vi "ConstellationRead.vi"(8 "error in":errorcluster, 9 "Active Boards":cluster{"Status":bool, "Board":string}[][](array[cluster]), 10 "Active Controllers":cluster{"Status":bool, "Number":dbl}[](array[cluster])=[{"Status"=TRUE, "Number"=0.0}, {"Status"=FALSE, "Number"=1.0}], 11 "Task in":refnum<visa-resource-name>[](array[refnum])) -> (0 "error out":errorcluster={"status"=FALSE, "code"=1073676294, "source"="VISA Read in ConstellationRead.vi->ConstellationTest.vi"}, 2 "Measurements":T1(array[cluster]), 3 "Task out":refnum<visa-resource-name>[](array[refnum]))   [LabVIEW 2012]
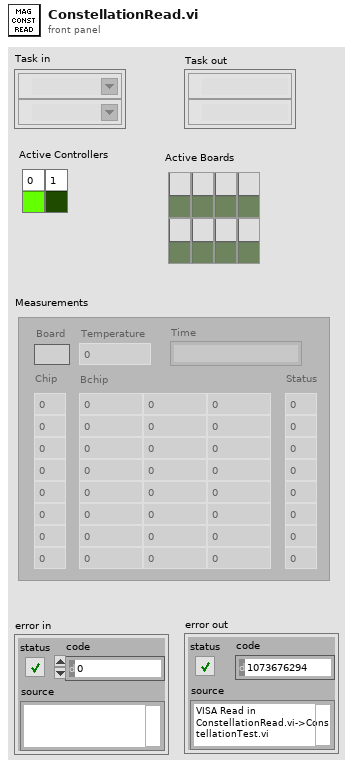
[diagram p1: front panel]
types:
  T1 = cluster{"Bchip":dbl[][], "Status":dbl[], "Temperature":dbl, "Chip":dbl[], "Board":string, "Time":string}[]
  T2 = cluster{"Bchip":dbl[][], "Status":dbl[], "Temperature":dbl, "Chip":dbl[], "Board":string, "Time Stamp":string}[]
  T3 = cluster{"Bchip":dbl[][], "Status":dbl[], "Temperature":dbl, "Chip":dbl[], "Board":string, "Time":string}
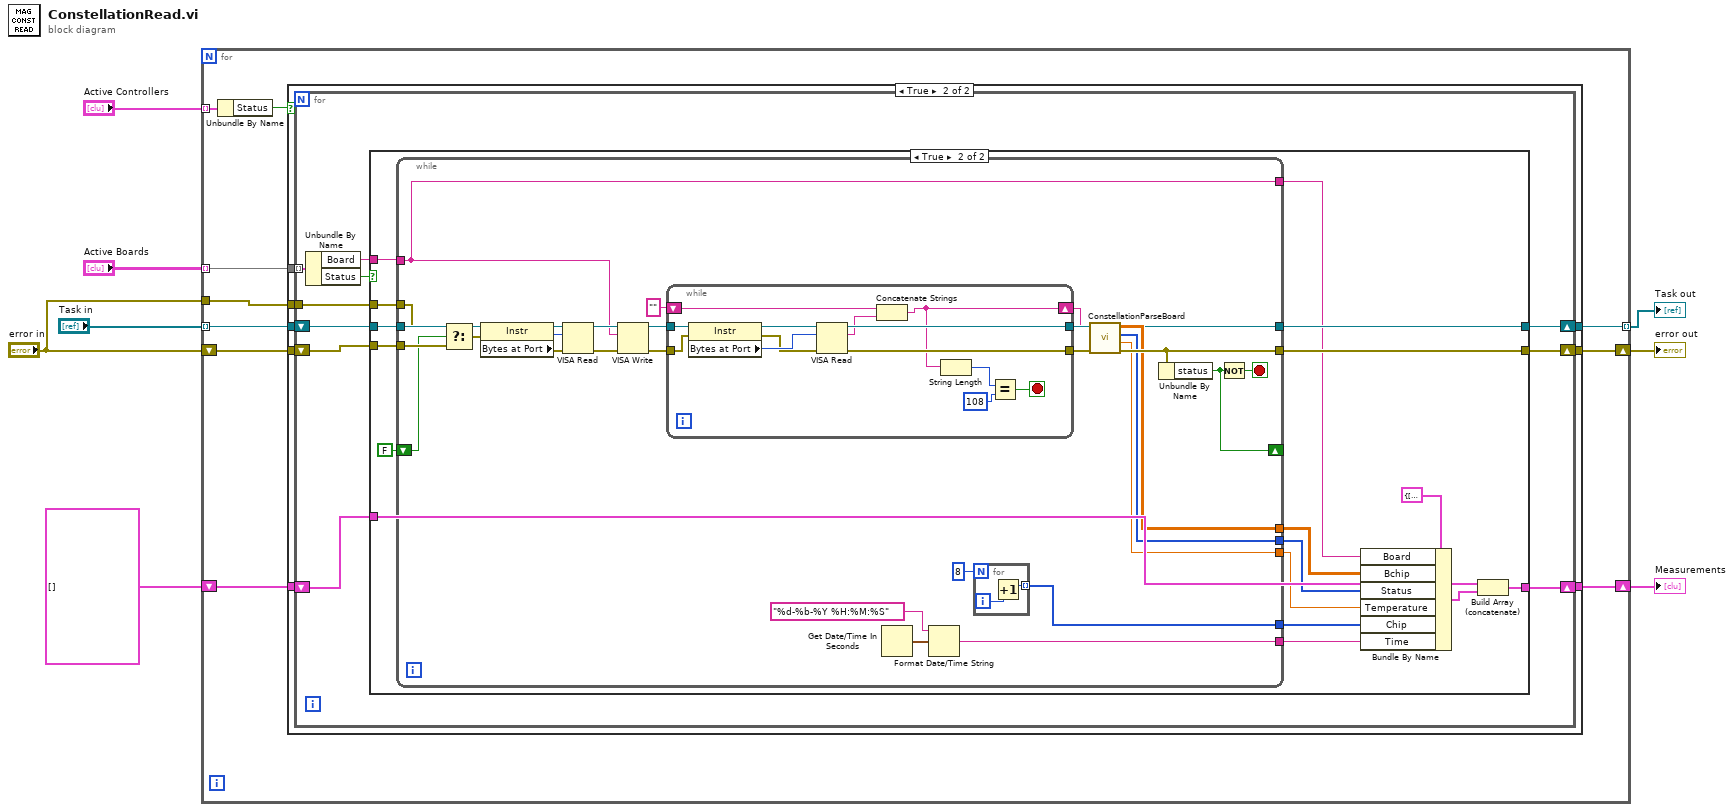
[diagram p0: block diagram]
diagram:
  n1 = for {
    tunnel: "Task in" -> [w16] mode=indexing
    tunnel: [w18] -> w6 mode=indexing
    shift-right: [w17] -> w7
    shift-left: "error in" -> [w15]
    tunnel: "error in" -> [w14]
    tunnel: "Active Controllers" -> [w13] mode=indexing
    shift-right: [w11] -> w3
    shift-left: T2 [] ("Measurements 2") -> [w10]
    tunnel: "Active Boards" -> [w9] mode=indexing
    n2 = Unbundle By Name(w13) -> ("Status"=w12:bool)
    n3 = case shown="True" w12 {
      tunnel: [w21 w29] -> w18
      tunnel: [w20 w28] -> w17
      tunnel: w16 -> [w21 w27]
      tunnel: w15 -> [w20 w26]
      tunnel: w14 -> [_ w25]
      tunnel: [w19 w24] -> w11
      tunnel: w10 -> [w19 w23]
      tunnel: w9 -> [_ w22]
      frame False {
      }
      frame True {
        n4 = for {
          shift-right: [w33] -> w29
          shift-left: w27 -> [w39]
          shift-right: [w34] -> w28
          shift-left: w26 -> [w38]
          tunnel: w25 -> [w37]
          shift-right: [w31] -> w24
          shift-left: w23 -> [w32]
          tunnel: w22 -> [w30] mode=indexing
          n5 = Unbundle By Name(w30) -> ("Board"=w36:string, "Status"=w35:bool)
          n6 = case shown="True" w35 {
            tunnel: w39 -> [w42 w59]
            tunnel: w38 -> [w41 w58]
            tunnel: w37 -> [_ w56]
            tunnel: w36 -> [_ w55]
            tunnel: [w41 w54] -> w34
            tunnel: [w42 w53] -> w33
            tunnel: w32 -> [w40 w52]
            tunnel: [w40 w51] -> w31
            frame False {
            }
            frame True {
              n7 = while {
                tunnel: w55 -> [w70]
                tunnel: [w66] -> w53
                tunnel: w59 -> [w87]
                tunnel: w58 -> [w63]
                tunnel: [w75] -> w54
                shift-right: [w71] -> _
                shift-left: FALSE ("status") -> [w60]
                tunnel: w56 -> [w62]
                tunnel: [w70] -> w50
                tunnel: [w74] -> w49
                tunnel: [w73] -> w48
                tunnel: [w72] -> w47
                tunnel: [w81] -> w46
                tunnel: [w78] -> w43
                stop <- w83 stop-if-true
                n8 = Select(t=w62, s=w60, f=w63) -> (s? t:f=w61:errorcluster)
                n9 = property class="Instr"(reference=w87, error in=w61) -> (reference out=w84:refnum<visa-resource-name>, error out=w85:errorcluster, "Bytes at Port"=w86:u32)
                n10 = VISA Read(VISA resource name=w84, byte count=w86, error in (no error)=w85) -> (VISA resource name out=w77:refnum<visa-resource-name>, error out=w76:errorcluster)  [unwired: 2 out]
                n11 = VISA Write(VISA resource name=w77, write buffer=w70, error in (no error)=w76) -> (VISA resource name out=w69:refnum<visa-resource-name>, error out=w68:errorcluster)  [unwired: 1 out]
                n12 = while {
                  tunnel: w69 -> [w100]
                  tunnel: [w92] -> w66
                  tunnel: w68 -> [w99]
                  tunnel: [w94] -> w67
                  shift-right: [w88] -> w65
                  shift-left: "" -> [w90]
                  stop <- w97 stop-if-true
                  n13 = property class="Instr"(reference=w100, error in=w99) -> (reference out=w93:refnum<visa-resource-name>, error out=w95:errorcluster, "Bytes at Port"=w96:u32)
                  n14 = VISA Read(VISA resource name=w93, byte count=w96, error in (no error)=w95) -> (VISA resource name out=w92:refnum<visa-resource-name>, read buffer=w91:string, error out=w94:errorcluster)  [unwired: 1 out]
                  n15 = Concatenate Strings(w90, w91) -> (w88:string)
                  n16 = String Length(string=w88) -> (length=w89:i32)
                  n17 = Equal?(x=w89, y=u32 108) -> (x = y?=w97:bool)
                }
                n18 = Get Date/Time In Seconds() -> (seconds since 1Jan1904=w80:timestamp)
                n19 = Format Date/Time String(time format string (%c)="%d-%b-%Y %H:%M:%S", seconds (now)=w80) -> (date/time string=w78:string)  [unwired: 1 in]
                n20 = for {
                  N: 8 -> [_]
                  tunnel: [w101] -> w81 mode=indexing
                  i -> [w102]
                  n21 = Increment(x=w102) -> (x+1=w101:i32)
                }
                n22 = call "ConstellationParseBoard.vi"("error in"=w67, "String"=w65) -> ("error out"=w75:errorcluster, "Temperature"=w72:sgl, "Status"=w73:i8[], "Bchip"=w74:sgl[][])  [unwired: 6 in]
                n23 = Unbundle By Name(w75) -> ("status"=w71:bool)
                n24 = Not(x=w71) -> (.not. x?=w83:bool)
              }
              n25 = Bundle By Name(cluster=T3 {"Bchip"=[[-0.1090909093618393, -0.44727271795272827, -0.18909090757369995], [-0.18272727727890015, -0.4272727370262146, -0.16363635659217834], [-0.23181818425655365, -0.3972727358341217, -0.2581818103790283], [-0.2754545509815216, -0.36000001430511475, -0.1963636428117752], [-0.32818183302879333, -0.3336363732814789, -0.23545454442501068], [-0.35181817412376404, -0.2645454406738281, -0.1645454615354538], [-0.12545454502105713, -0.44363635778427124, -0.24272727966308594], [-0.30636364221572876, -0.34454545378685, -0.17363636195659637]], "Status"=[1.0, 1.0, 1.0, 1.0, 1.0, 1.0, 1.0, 1.0], "Temperature"=1.4561904668807983, "Chip"=[1.0, 2.0, 3.0, 4.0, 5.0, 6.0, 7.0, 8.0], "Board"="A", "Time"="20-Nov-2015 11:26:39"} ("Board Measurement"), "Board"=w50, "Bchip"=w49, "Status"=w48, "Temperature"=w47, "Chip"=w46, "Time"=w43) -> (w45:T3)
              n26 = Build Array (concatenate)(w52, w45) -> (w51:T1)
            }
          }
        }
      }
    }
  }
  "error out" <- w7
  "Task out" <- w6
  "Measurements" <- w3
